vi "save_xml.vi"(8 "error in":errorcluster, 10 "All scan parameters":T1={"Fiber parameters"={"Frequency"=100.0, "Amplitude X"=0.0, "Amplitude Y"=0.0, "Initial Amplitude X"=0.0, "Initial Amplitude Y"=0.0, "Phase"=0.0}, "Spiral parameters"={"Imaging periods"=1.0, "Settling periods"=1.0, "Resting periods"=1.0}, "Run parameters"={"Run mode"=enum."Continuous", "Averages per frame"=1, "No. of frames"=1}, "Acquisition parameters"={"Cycles per pixel"=1, "Image size"=128}, "Fiber parameters pixel_mapper"={"Frequency"=100.0, "Amplitude X"=0.0, "Amplitude Y"=0.0, "Initial Amplitude X"=0.0, "Initial Amplitude Y"=0.0, "Phase"=0.0}, "Smooth_coeffs_cluster"={"Coeff 1"=0.0, "Coeff 2"=0.0}, "Storage parameters"={"Autosave"=FALSE, "Path"=path ""}} {"Smooth_coeffs_cluster"."Coeff 1" min=0.0 max=1.0 step=0.05; "Smooth_coeffs_cluster"."Coeff 2" min=0.0 max=1.0 step=0.05; "Fiber parameters pixel_mapper"."Phase" min=-90.0 max=90.0 step=5.0; "Fiber parameters pixel_mapper"."Initial Amplitude Y" min=0.0 max=1.0 step=0.1; "Fiber parameters pixel_mapper"."Initial Amplitude X" min=0.0 max=1.0 step=0.1; "Fiber parameters pixel_mapper"."Amplitude Y" min=0.0 max=3.0 step=0.1; "Fiber parameters pixel_mapper"."Amplitude X" min=0.0 max=3.0 step=0.1; "Fiber parameters pixel_mapper"."Frequency" min=100.0 max=6000.0 step=1.0; "Acquisition parameters"."Image size" items=["128x128 px"=128, "256x256 px"=256, "512x512 px"=512]; "Acquisition parameters"."Cycles per pixel" min=100 max=90000 step=1; "Run parameters"."No. of frames" min=1 max=1000 step=1; "Run parameters"."Averages per frame" min=1 max=32; "Spiral parameters"."Resting periods" min=10.0 max=1000.0 step=1.0; "Spiral parameters"."Settling periods" min=1.0 max=1000.0 step=1.0; "Spiral parameters"."Imaging periods" min=1.0 max=1000.0 step=1.0; "Fiber parameters"."Phase" min=-90.0 max=90.0 step=5.0; "Fiber parameters"."Initial Amplitude Y" min=0.0 max=1.0 step=0.1; "Fiber parameters"."Initial Amplitude X" min=0.0 max=1.0 step=0.1; "Fiber parameters"."Amplitude Y" min=0.0 max=3.0 step=0.1; "Fiber parameters"."Amplitude X" min=0.0 max=3.0 step=0.1; "Fiber parameters"."Frequency" min=100.0 max=6000.0 step=1.0}, 11 "Path":string) -> (0 "error out":errorcluster)   [LabVIEW 2011, in "Fiberscope_library.lvlib"]
uses:
  Fiberscope_library.lvlib
  typedefs/all_scan_parameters_cluster.ctl
  typedefs/fiber_parameters_cluster.ctl
  typedefs/spiral_parameters_cluster.ctl
  typedefs/run_parameters_cluster.ctl
  typedefs/run_mode_enum.ctl
  typedefs/acquisition_parameters_cluster.ctl
  typedefs/image_size_I32.ctl
  typedefs/smooth_coeffs_cluster.ctl
  typedefs/storage_parameters_cluster.ctl
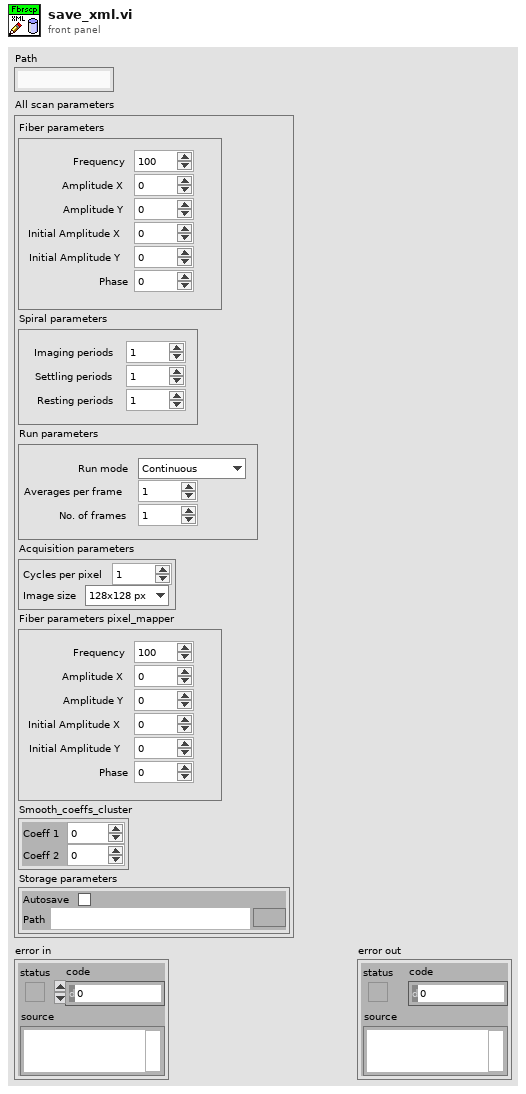
[diagram p1: front panel]
types:
  T1 = typedef "Fiberscope_library.lvlib/all_scan_parameters_cluster.ctl" = cluster{"Fiber parameters":T2, "Spiral parameters":T3, "Run parameters":T4, "Acquisition parameters":T6, "Fiber parameters pixel_mapper":T2, "Smooth_coeffs_cluster":T8, "Storage parameters":T9}
  T2 = typedef "Fiberscope_library.lvlib/fiber_parameters_cluster.ctl" = cluster{"Frequency":dbl, "Amplitude X":dbl, "Amplitude Y":dbl, "Initial Amplitude X":dbl, "Initial Amplitude Y":dbl, "Phase":dbl}
  T3 = typedef "Fiberscope_library.lvlib/spiral_parameters_cluster.ctl" = cluster{"Imaging periods":dbl, "Settling periods":dbl, "Resting periods":dbl}
  T4 = typedef "Fiberscope_library.lvlib/run_parameters_cluster.ctl" = cluster{"Run mode":T5, "Averages per frame":u8, "No. of frames":u32}
  T5 = typedef "Fiberscope_library.lvlib/run_mode_enum.ctl" = enum16{"Continuous", "Single frame", "No. of frames"}
  T6 = typedef "Fiberscope_library.lvlib/acquisition_parameters_cluster.ctl" = cluster{"Cycles per pixel":u32, "Image size":T7}
  T7 = typedef "Fiberscope_library.lvlib/image_size_I32.ctl" = i32
  T8 = typedef "Fiberscope_library.lvlib/smooth_coeffs_cluster.ctl" = cluster{"Coeff 1":dbl, "Coeff 2":dbl}
  T9 = typedef "Fiberscope_library.lvlib/storage_parameters_cluster.ctl" = cluster{"Autosave":bool, "Path":path}
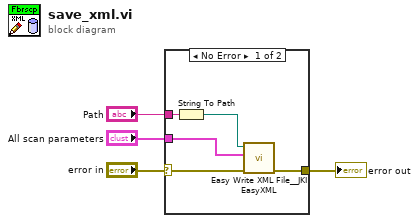
[diagram p0: block diagram]
diagram:
  n1 = case shown="No Error" "error in" {
    selector: "error in" -> [w8 w10]
    tunnel: [w7 w10] -> w3
    tunnel: "Path" -> [w9 _]
    tunnel: "All scan parameters" -> [w5 _]
    frame No Error {
      n2 = String To Path(string=w9) -> (path=w6:path)
      n3 = call <vilib>:"Easy Write XML File__JKI EasyXML.vi"("error in (no error)"=w8, "LabVIEW Data"=w5, "XML File Path"=w6) -> ("error out"=w7:errorcluster)  [unwired: 7 in, 1 out]
    }
    frame Error {
    }
  }
  "error out" <- w3
